vi "Obtain Report.vi"(8 "error in (no error)":errorcluster, 11 "Execution in":refnum<class "Execution.lvclass">) -> (0 "error out":errorcluster, 2 "Report":refnum<class "Report.lvclass">, 3 "Execution out":refnum<class "Execution.lvclass">)   [LabVIEW 2020, in "TSnax.lvlib" / "Execution.lvclass"]
uses:
  Execution.lvclass
  Execution.lvclass/Execution.ctl
  Engine/Engine.lvclass
  Report/Report.lvclass
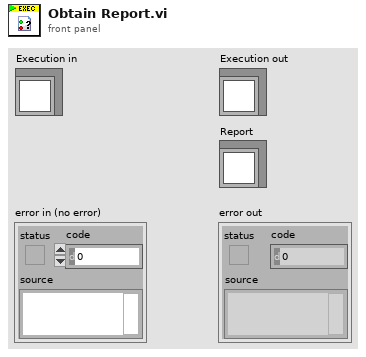
[diagram p1: front panel]
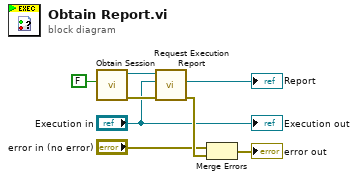
[diagram p0: block diagram]
diagram:
  n1 = call "Obtain Session.vi"("Create if needed? (T)"=FALSE) -> ("error out"=w4:errorcluster, "Engine out"=w5:refnum<class "Engine.lvclass">)  [unwired: 9 in]
  n2 = call "Request Execution Report.vi"("error in (no error)"=w4, "Execution"="Execution in", "Engine in"=w5) -> ("error out"=w8:errorcluster, "Report"=→"Report":refnum<class "Report.lvclass">)  [unwired: 6 in, 1 out]
  n3 = Merge Errors("error in (no error)", w8) -> (→"error out":errorcluster)
  "Execution out" <- "Execution in"
